vi "buttonVisibility.vi"(8 "error in":errorcluster, 9 "reference":refnum<vi>, 10 "Button Refs":refnum<vi>[](array[refnum]), 11 "Data in":T1={"Report.lvclass"=refnum, "Norm"="", "last State"=enum."Initialize", "Norm ID"=0, "EMTestCWS500N.lvclass"=refnum, "CEG4500.lvclass"=refnum, "Tektronix RSA5106A.lvclass"=refnum, "erfolgreich"=FALSE, "Device Enum"=enum."emTestCWS500N", "Test Enum"=enum."ESD", "debug"=FALSE, "tab"=enum."Hauptmenü", "ESD Pistol.lvclass"=refnum, "SubPnl Refnum"=refnum, "TabCtl Refnum"=refnum, "ButtonsEinblenden?"=FALSE, "VKey"=enum."ASCII", "last Test"=refnum, "Class 4.lvclass"=refnum}) -> (0 "error out":errorcluster, 3 "Data out":T1={"Report.lvclass"=refnum, "Norm"="", "last State"=enum."Initialize", "Norm ID"=0, "EMTestCWS500N.lvclass"=refnum, "CEG4500.lvclass"=refnum, "Tektronix RSA5106A.lvclass"=refnum, "erfolgreich"=FALSE, "Device Enum"=enum."emTestCWS500N", "Test Enum"=enum."ESD", "debug"=FALSE, "tab"=enum."Hauptmenü", "ESD Pistol.lvclass"=refnum, "SubPnl Refnum"=refnum, "TabCtl Refnum"=refnum, "ButtonsEinblenden?"=FALSE, "VKey"=enum."ASCII", "last Test"=refnum, "Class 4.lvclass"=refnum})   [LabVIEW 2013, in "Utilities.lvlib"]
uses:
  lib/Utilities.lvlib
  Main/controls/Data.ctl
  classes/Datastructure/Report/Report.lvclass
  classes/Devices/emTestCWS500N/EMTestCWS500N.lvclass
  classes/Devices/CEG4500/CEG4500.lvclass
  classes/Devices/Tektronix RSA5106A/Tektronix RSA5106A.lvclass
  ESD Pistol.lvclass
  classes/Datastructure/Test/Test.lvclass
  classes/Devices/Class4/Class 4.lvclass
  Main/controls/State.ctl
  classes/Devices/DeviceInterface/Devices.ctl
  classes/Tests/TestInterface/Tests.ctl
  Tabs.ctl
  <vilib>/event_ctls.llb/eventvkey.ctl
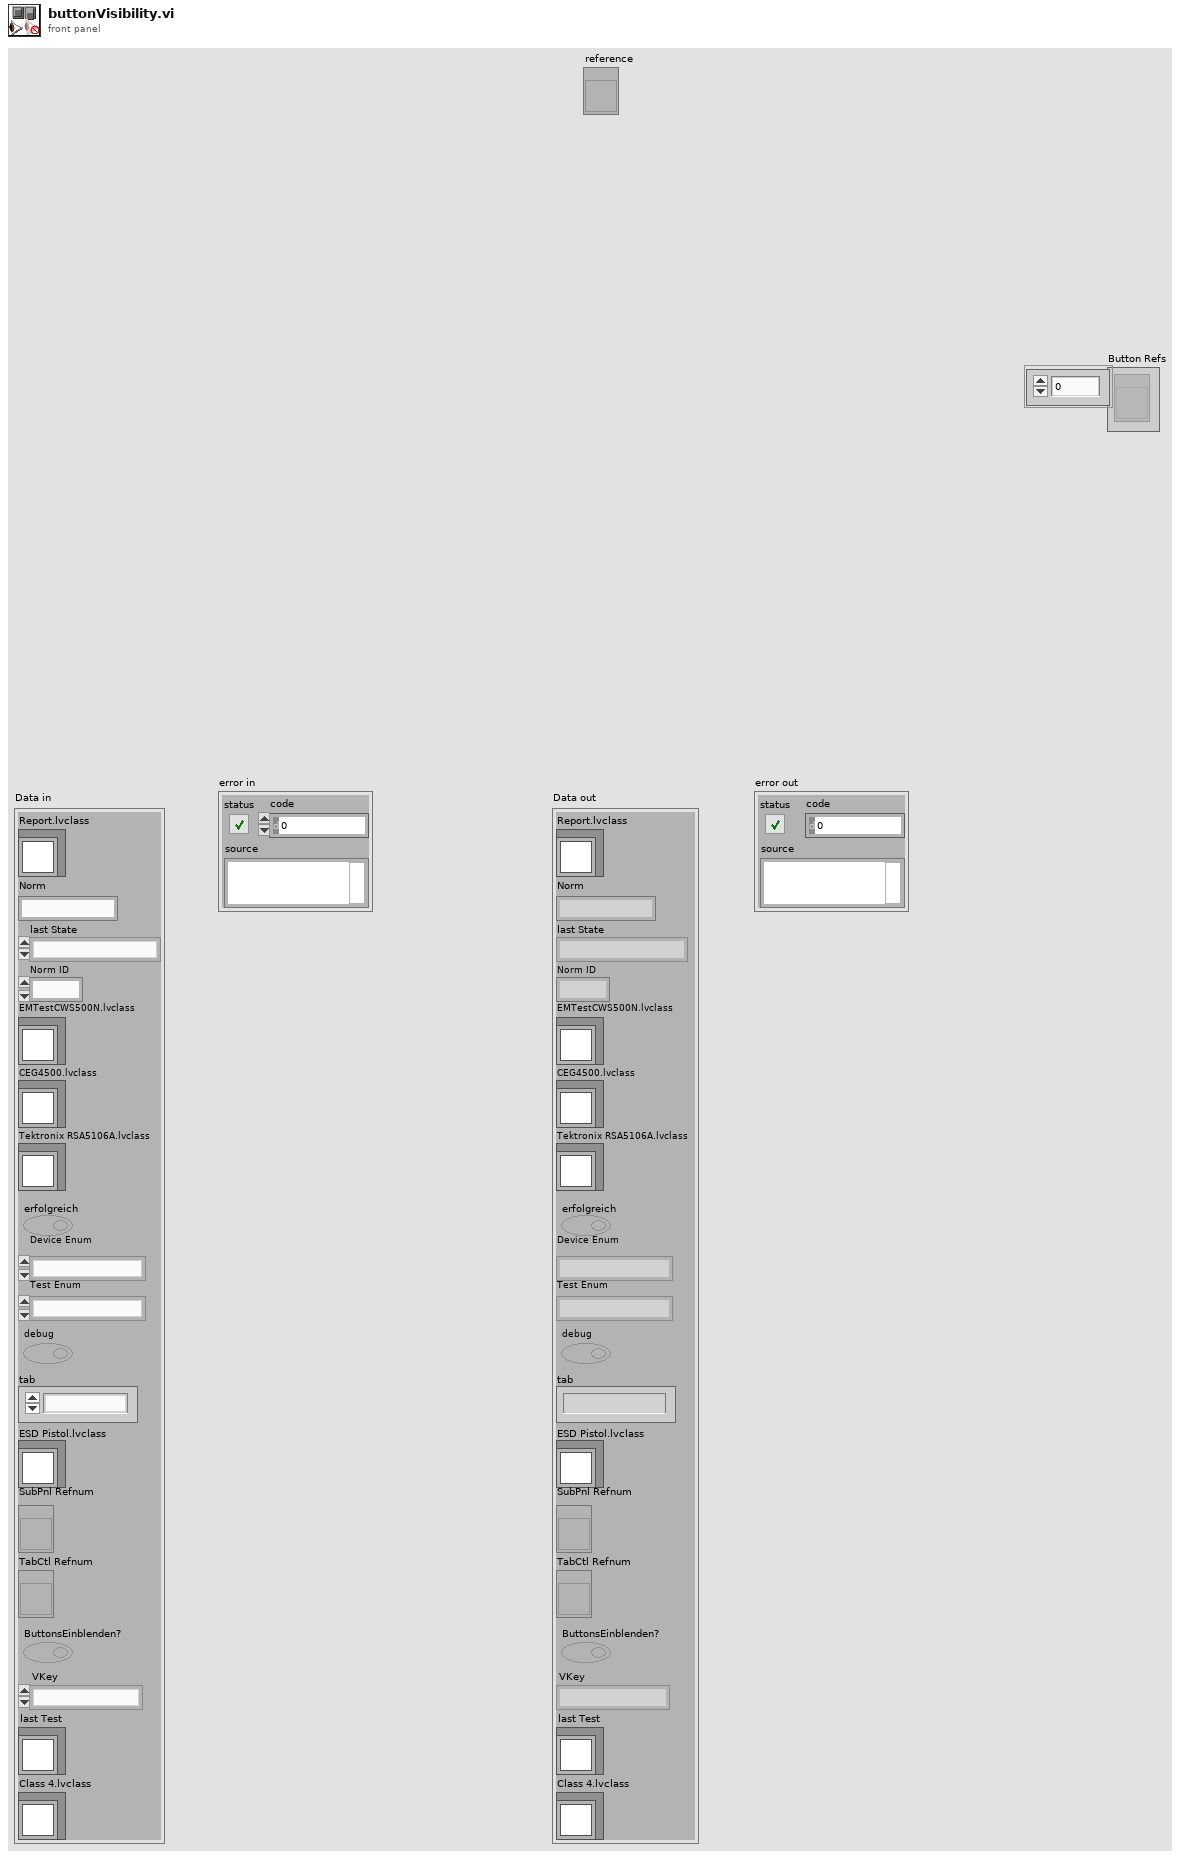
[diagram p1: front panel]
types:
  T1 = typedef "Data.ctl" = cluster{"Report.lvclass":refnum<class "Report.lvclass">, "Norm":string, "last State":T2, "Norm ID":i32, "EMTestCWS500N.lvclass":refnum<class "EMTestCWS500N.lvclass">, "CEG4500.lvclass":refnum<class "CEG4500.lvclass">, "Tektronix RSA5106A.lvclass":refnum<class "Tektronix RSA5106A.lvclass">, "erfolgreich":bool, "Device Enum":T3, "Test Enum":T4, "debug":bool, "tab":T5, "ESD Pistol.lvclass":refnum<class "ESD Pistol.lvclass">, "SubPnl Refnum":refnum<vi>, "TabCtl Refnum":refnum<vi>, "ButtonsEinblenden?":bool, "VKey":T6, "last Test":refnum<class "Test.lvclass">, "Class 4.lvclass":refnum<class "Class 4.lvclass">}
  T2 = typedef "State.ctl" = enum16{"create Pdf", "edit Report", "load Report", "save Report", "do Test", "CDN Kalibrierung", "enter Report Parameters", "new Test", "Protokoll", "read Tree", "update Tree", "Fehler", "Initialize", "Wait for Event", "Exit"}
  T3 = typedef "Devices.ctl" = enum16{"unbekannt", "ESD Pistol", "Tektronix RSA5106A", "emTestCWS500N", "CEG-4500"}
  T4 = typedef "Tests.ctl" = enum16{"unbekannt", "Störaussendung", "Burst", "ESD", "Surge", "Spannungseinbruch", "HF-Felder"}
  T5 = typedef "Tabs.ctl" = enum32{"Hauptmenü", "Prüfbericht", "Einstellungen"}
  T6 = typedef "eventvkey.ctl" = enum16{"ASCII", "Enter", "Return", "Shift", "Ctrl", "Alt", "Cmd", "Opt", "Caps", "NumLock", "Clear", "Break", "Up", "Down", "Left", "Right", "Insert", "Delete", "Home", "End", "PageUp", "PageDown", "Escape", "Help", "Pause", "ScrollLock", "F1", "F2", "F3", "F4", "F5", "F6", "F7", "F8", "F9", "F10", "F11", "F12", "F13", "F14", "F15", "F16", "F17", "F18", "F19", "F20", "F21", "F22", "F23", "F24", "Play", "VolumeUp", "VolumeDown", "Mute", "Two Byte Char"}
  T7 = enum8{"Enabled", "Disabled", "Disabled and Grayed Out"}
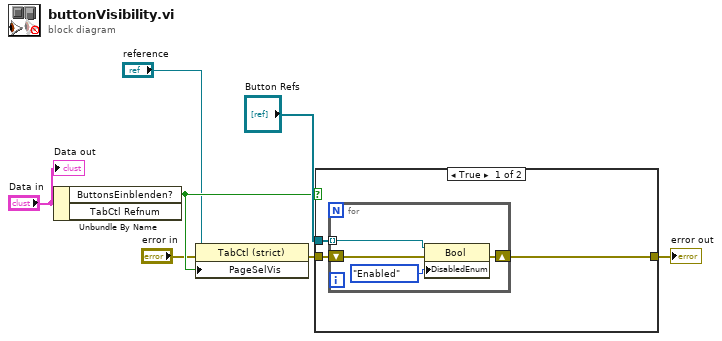
[diagram p0: block diagram]
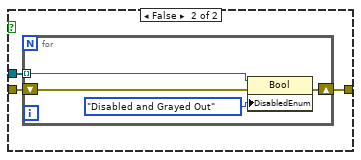
[diagram p2: hidden frame]
diagram:
  n1 = Unbundle By Name("Data in") -> ("ButtonsEinblenden?"=w4:bool)  [unwired: 1 out]
  n2 = property class="TabCtl (strict)"(reference="reference", error in="error in", "PageSelVis"=w4) -> (error out=w5:errorcluster)  [unwired: 1 out]
  n3 = case shown="True" w4 {
    tunnel: "Button Refs" -> [w10 w17]
    tunnel: w5 -> [w9 w16]
    tunnel: [w8 w15] -> w2
    frame True {
      n4 = for {
        shift-right: [w12] -> w8
        shift-left: w9 -> [w14]
        tunnel: w10 -> [w13] mode=indexing
        n5 = property class="Bool"(reference=w13, error in=w14, "DisabledEnum"=T7."Enabled" ("Deaktiviert")) -> (error out=w12:errorcluster)  [unwired: 1 out]
      }
    }
    frame False {
      n6 = for {
        shift-right: [w19] -> w15
        shift-left: w16 -> [w21]
        tunnel: w17 -> [w20] mode=indexing
        n7 = property class="Bool"(reference=w20, error in=w21, "DisabledEnum"=T7."Disabled and Grayed Out" ("Deaktiviert")) -> (error out=w19:errorcluster)  [unwired: 1 out]
      }
    }
  }
  "error out" <- w2
  "Data out" <- "Data in"
